vi "settingsEventsFunctionalGlobal.vi"(9 "settingsEvents":T1, 11 "Action":enum16{"Write", "Read"}(ring)) -> (1 "settingsEvents":T1)   [LabVIEW 2011, in "Tools.lvlib" / "Settings.lvlib"]
doc: "This vi makes Settings Manager Events available globally via the SettingsEventsManager.\nThe SettingsEventsManager must be used to access the events."
uses:
  Settings.lvlib
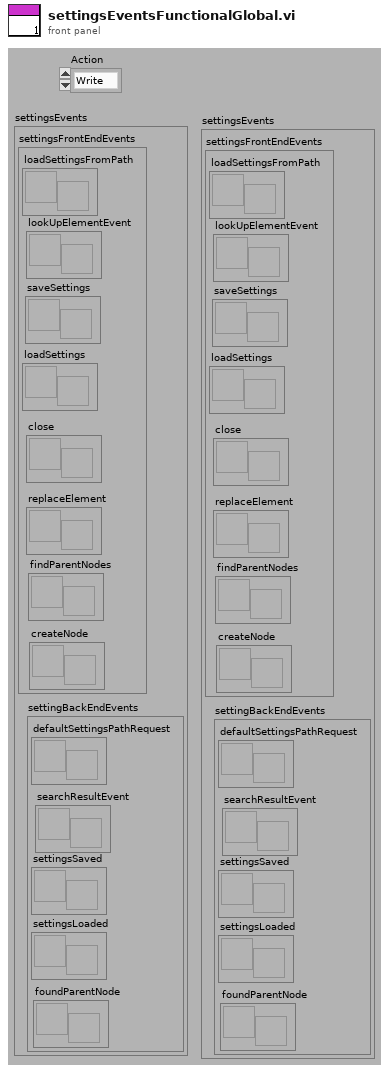
[diagram p1: front panel]
types:
  T1 = cluster{"settingsFrontEndEvents":cluster{"loadSettingsFromPath":refnum<user-event>, "lookUpElementEvent":refnum<user-event>, "saveSettings":refnum<user-event>, "loadSettings":refnum<user-event>, "close":refnum<user-event>, "replaceElement":refnum<user-event>, "findParentNodes":refnum<user-event>, "createNode":refnum<user-event>}, "settingBackEndEvents":cluster{"defaultSettingsPathRequest":refnum<user-event>, "searchResultEvent":refnum<user-event>, "settingsSaved":refnum<user-event>, "settingsLoaded":refnum<user-event>, "foundParentNode":refnum<user-event>}}
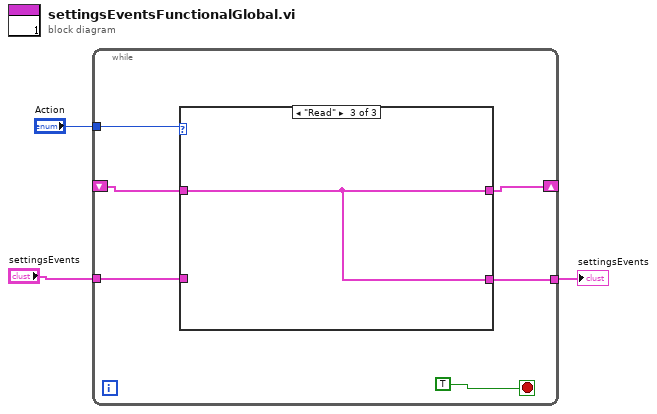
[diagram p0: block diagram]
diagram:
  n1 = while {
    tunnel: "Action" -> [w9]
    shift-right: [w4] -> _
    shift-left: _ -> [w6]
    tunnel: "settingsEvents" -> [w7]
    tunnel: [w5] -> w1
    stop <- TRUE stop-if-true
    n2 = case shown="\"Read\"" w9 {
      tunnel: [w11 w12 w13] -> w4
      tunnel: w7 -> [w10 w12 _]
      tunnel: w6 -> [w11 _ w13]
      tunnel: [w10 w12 w13] -> w5
      frame Default {
      }
      frame "Write" {
      }
      frame "Read" {
      }
    }
  }
  "settingsEvents" <- w1
